vi "Analog Voltage DAQ Setup.vi"(0 "physical channels":tag, 1 "sample mode":i32(ring)=10123 items=["Finite Samples"=10178, "Continuous Samples"=10123, "Hardware Timed Single Point"=12522], 2 "error in":errorcluster, 3 "input terminal configuration":i32(ring)=10083 items=["Default"=-1, "RSE"=10083, "NRSE"=10078, "Differential"=10106, "Pseudodifferential"=12529], 5 "Sample Rate":dbl=1000.0 format="%0.2f", 7 "task in":refnum<k21>, 9 "minimum value":dbl format="%0.2f", 11 "maximum value":dbl=1.0 format="%0.2f", 12 "samples per channel":i32=1) -> (4 "task out":refnum<k21>, 15 "error out":errorcluster)   [LabVIEW 2016]
uses:
  <vilib>/DAQmx/create/channels.llb/DAQmx Create Channel (AI-Voltage-Basic).vi
  <vilib>/DAQmx/configure/timing.llb/DAQmx Timing (Sample Clock).vi
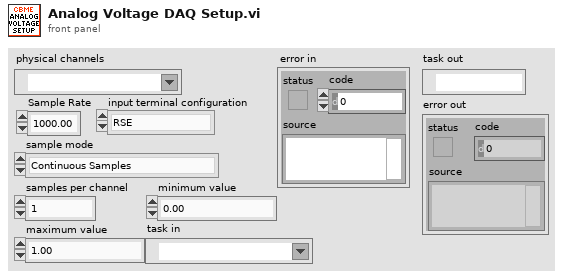
[diagram p1: front panel]
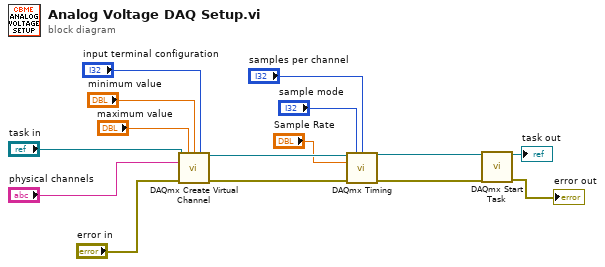
[diagram p0: block diagram]
diagram:
  n1 = call-poly <vilib>:"DAQmx Create Virtual Channel.vi"("task in"="task in", "maximum value"="maximum value", "minimum value"="minimum value", "input terminal configuration"="input terminal configuration", "physical channels"="physical channels", "error in"="error in") -> ("task out"=w14:refnum<k21>, "error out"=w10:errorcluster)  [unwired: 8 in]
  n2 = call-poly <vilib>:"DAQmx Timing.vi"("task/channels in"=w14, "sample mode"="sample mode", "samples per channel"="samples per channel", "rate"="Sample Rate", "error in"=w10) -> ("task out"=w9:refnum<k21>, "error out"=w8:errorcluster)  [unwired: 9 in]
  n3 = call <vilib>:"DAQmx Start Task.vi"("task/channels in"=w9, "error in"=w8) -> ("task out"=→"task out":refnum<k21>, "error out"=→"error out":errorcluster)  [unwired: 12 in]
